vi "FormulaSqrt.vi"() -> ()   [LabVIEW 2025]
panel:
  out "Result":dbl
  in  "Number":dbl
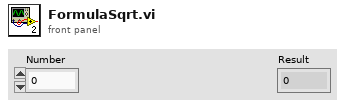
[diagram p1: front panel]
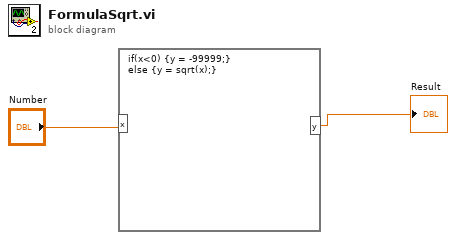
[diagram p0: block diagram]
diagram:
  n1 = formula code="if(x<0) {y = -99999;}\nelse {y = sqrt(x);}"("x"="Number") -> ("y"=→"Result":dbl)
